vi "JKISM++ Running Log - DebugTool.vi"() -> ()   [LabVIEW 2014]
uses:
  _Support/GlobalEvent/FGV-GlobalEventRef.vi
  JKI-State-Machine-Plus.lvlib
panel:
  out "State History":string
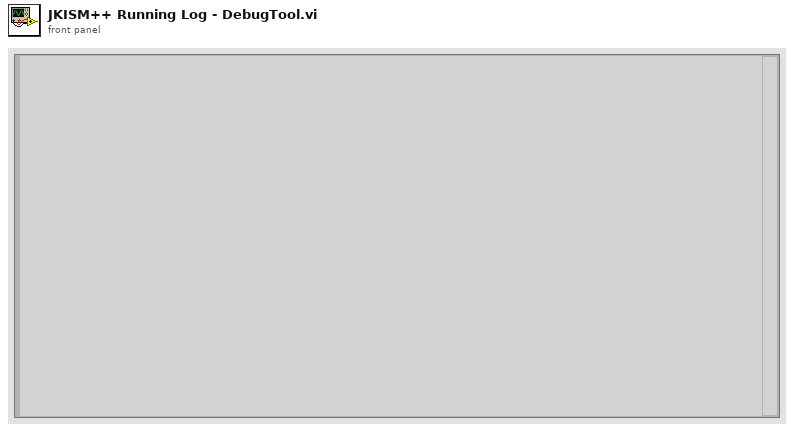
[diagram p1: front panel]
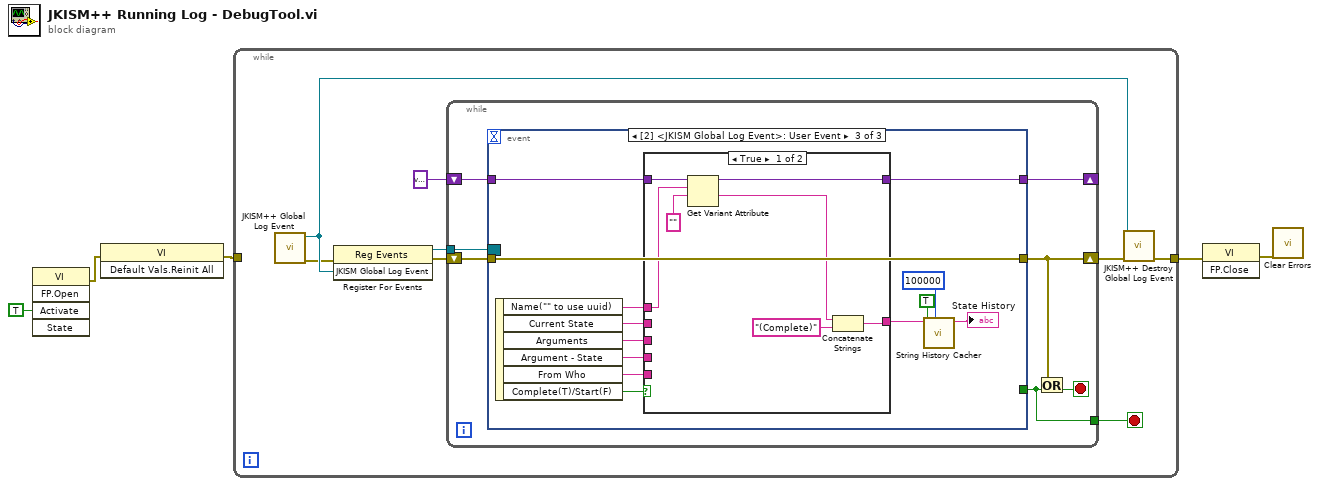
[diagram p0: block diagram]
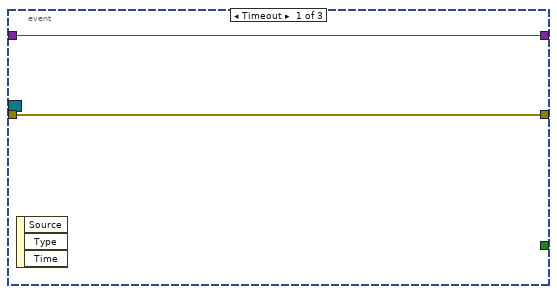
[diagram p2: hidden frame]
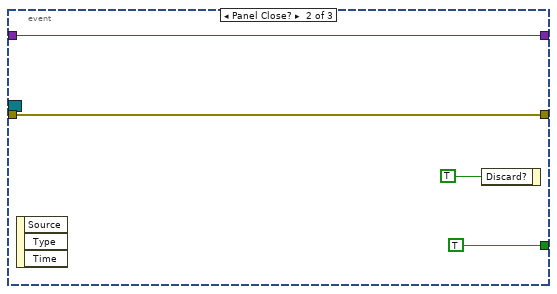
[diagram p3: hidden frame]
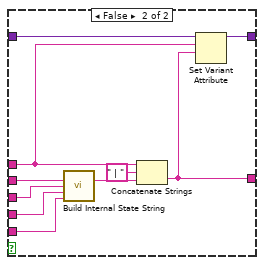
[diagram p4: hidden frame]
diagram:
  n1 = invoke class="VI" method="FP.Open"("Activate"=TRUE ("Activate?")) -> (error out=w4:errorcluster)  [unwired: 4 in, 4 out]
  n2 = invoke class="VI" method="Default Vals.Reinit All"(error in=w4) -> (error out=w3:errorcluster)  [unwired: 2 in, 2 out]
  n3 = while {
    tunnel: w3 -> [_]
    tunnel: [w7] -> w2
    stop <- w8 stop-if-true
    n4 = call "JKISM++ Global Log Event.vi"() -> ("Error out"=w9:errorcluster, "JKISM Global Log Event"=w10:refnum<user-event>)  [unwired: 10 in]
    n5 = register-events(error in=w9, w10) -> (reference out=w13:refnum<event-registration>, error out=w12:errorcluster)  [unwired: 1 in]
    n6 = while {
      tunnel: w13 -> [w20]
      shift-right: [w17] -> w11
      shift-left: w12 -> [w19]
      tunnel: [w16] -> w8
      shift-right: [w14] -> _
      shift-left: variant -> [w15]
      stop <- w18 stop-if-true
      n7 = event shown="[2] <JKISM Global Log Event>: User Event" {
        selector: w20 -> [_ _ _]
        dyn-events: _ -> [_ _ _]
        timeout: _ -> [_ _ _]
        tunnel: w19 -> [w22 w26 w39]
        tunnel: [w22 w26 w39] -> w17
        tunnel: [_ TRUE ("Discard?") _] -> w16
        tunnel: w15 -> [w21 w23 w31]
        tunnel: [w21 w23 w30] -> w14
        event Timeout {
          n8 = event-data() -> ()  [unwired: 1 in, 3 out]
        }
        event Panel Close? {
          n9 = event-data() -> ()  [unwired: 1 in, 3 out]
          n10 = event-data("Discard?"=TRUE) -> ()  [unwired: 1 in, 1 out]
        }
        event User Event {
          n11 = event-data() -> ("Name(\"\" to use uuid)"=w29:string, "Current State"=w36:string, "Arguments"=w35:string, "Argument - State"=w34:string, "From Who"=w33:string, "Complete(T)/Start(F)"=w27:bool)  [unwired: 1 in]
          n12 = case shown="True" w27 {
            tunnel: w36 -> [_ w55]
            tunnel: w35 -> [_ w54]
            tunnel: w34 -> [_ w53]
            tunnel: w33 -> [_ w52]
            tunnel: w31 -> [w46 w50]
            tunnel: [w45 w49] -> w30
            tunnel: w29 -> [w44 w48]
            tunnel: [w42 w47] -> w28
            frame True {
              n13 = Get Variant Attribute(Variant=w46, name=w44, default value (empty Variant)="") -> (duplicate Variant=w45:variant, value=w41:string)  [unwired: 1 in, 2 out]
              n14 = Concatenate Strings(w41, "(Complete)" ("string")) -> (w42:string)
            }
            frame False {
              n15 = call "Build Internal State String.vi"("State"=w55, "Arguments (\"\")"=w54, "Arg-State (\"\")"=w53, "Source (\"\")"=w52) -> ("State with Arguments"=w56:string)  [unwired: 11 in]
              n16 = Concatenate Strings(w48, " | " ("string"), w56) -> (w47:string)
              n17 = Set Variant Attribute(Variant=w50, name=w48, value=w47) -> (Variant out=w49:variant)  [unwired: 1 in, 2 out]
            }
          }
          n18 = call "String History Cacher.vi"("length"=100000, "Include Timestamp(F)"=TRUE, "String"=w28) -> ("String Cache"=→"State History":string)  [unwired: 8 in]
        }
      }
      n19 = Or(x=w17, y=w16) -> (x .or. y?=w18:bool)
    }
    n20 = call "JKISM++ Destroy Global Log Event.vi"("Error in"=w11, "JKISM Global Log Event"=w10) -> ("Error out"=w7:errorcluster)  [unwired: 9 in]
  }
  n21 = invoke class="VI" method="FP.Close"(error in=w2) -> (error out=w1:errorcluster)  [unwired: 2 in, 2 out]
  n22 = call <vilib>:"Clear Errors.vi"("error in (no error)"=w1) -> ()  [unwired: 6 in, 1 out]
